vi "rs3 Advanced set SLO Threshold3.vi"(8 "error in (no error)":errorcluster, 10 "ST SLO Threshold":T1, 11 "device in":u64) -> (0 "error out":errorcluster, 1 "error":u64, 3 "Dev out":u64)   [LabVIEW 2019, in "libRealSense3.lvlib"]
doc: "This sets some registers that affect the depth calculations"
uses:
  libRealSense3.lvlib
  realsense2.dll
panel:
  # "RS3 Adv. Set SLO Threshold 2"
  # "(C) 2017 Intel Corp.,  AGJ"
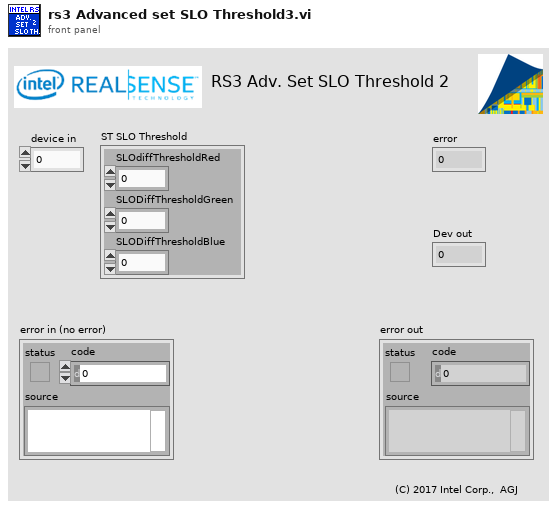
[diagram p1: front panel]
types:
  T1 = cluster{"SLOdiffThresholdRed":u32, "SLODiffThresholdGreen":u32, "SLODiffThresholdBlue":u32}
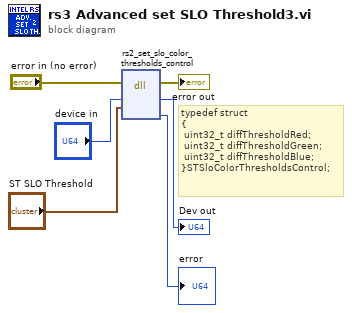
[diagram p0: block diagram]
diagram:
  # "typedef struct\n{\n\tuint32_t diffThresholdRed;\n\tuint32_t diffThresholdGreen;\n\tuint32_t diffThresholdBlue;\n}STSloColorThresholdsControl;"
  n1 = dll-call lib="C:/Users/morte/Documents/gitmoro/treadmill/RealSense for Labview ver. 2.33/realsense2.dll" fn="rs2_set_slo_color_thresholds_control"(error in="error in (no error)", "device"="device in", "ST SLO Threshold"="ST SLO Threshold") -> (error out=→"error out":errorcluster, "device"=→"Dev out":u64, "error"=→"error":u64)  [unwired: 5 in, 1 out]
